vi "Configure Hardware r2.vi"(7 "DAQmx Cluster In":T1 {"ai DAQmx Cluster"."input terminal configuration" items=["Default"=-1, "RSE"=10083, "NRSE"=10078, "Differential"=10106, "Pseudodifferential"=12529]; "bc DAQmx Cluster"."Scaling Information"."electrical units" items=["Volts/Volt"=15896, "mVolts/Volt"=15897]; "bc DAQmx Cluster"."Scaling Information"."physical units" items=["Newtons"=15875, "Pounds"=15876, "kgf"=15877]; "bc DAQmx Cluster"."Bridge Information"."bridge configuration" items=["Full Bridge"=10182, "Half Bridge"=10187, "Quarter Bridge"=10270]; "bc DAQmx Cluster"."Bridge Information"."voltage excitation source" items=["Internal"=10200, "External"=10167]; "tc DAQmx Cluster"."Thermocouple Type" items=["J"=10072, "K"=10073, "N"=10077, "R"=10082, "S"=10085, "T"=10086, "B"=10047, "E"=10055]; "tc DAQmx Cluster"."Units" items=["Deg C"=10143, "Deg F"=10144, "Kelvins"=10325, "Deg R"=10145, "From Custom Scale"=10065]}, 8 "error in (no error)":errorcluster, 11 "DAQmx Container In":T2) -> (0 "error out":errorcluster, 3 "DAQmx Container Out":T2)   [LabVIEW 2024]
doc: "Configure the hardware."
uses:
  support/Control/DAQmx Container.ctl
  Configuration/DAQmx Configuration.ctl
  <vilib>/DAQmx/create/channels.llb/DAQmx Create Channel (DO-Digital Output).vi
  <vilib>/DAQmx/create/channels.llb/DAQmx Create Channel (AI-Force-Bridge-Two-Point-Linear).vi
  <vilib>/DAQmx/configure/timing.llb/DAQmx Timing (Sample Clock).vi
  <vilib>/DAQmx/create/channels.llb/DAQmx Create Channel (AI-Voltage-Basic).vi
  <vilib>/DAQmx/create/channels.llb/DAQmx Create Channel (AI-Temperature-Thermocouple).vi
  <vilib>/DAQmx/create/channels.llb/DAQmx Create Channel (DI-Digital Input).vi
  <resource>/objmgr/daqmx.rc
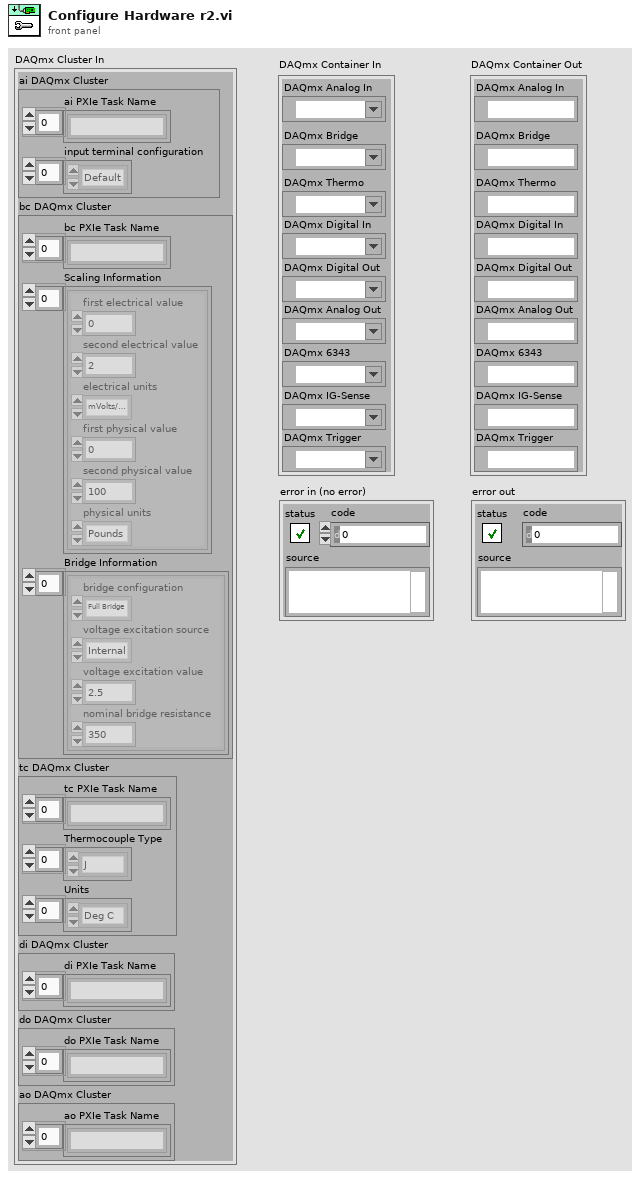
[diagram p1: front panel]
types:
  T1 = typedef "DAQmx Configuration.ctl" = cluster{"ai DAQmx Cluster":cluster{"ai PXIe Task Name":string[], "input terminal configuration":i32[]}, "bc DAQmx Cluster":cluster{"bc PXIe Task Name":string[], "Scaling Information":cluster{"first electrical value":dbl, "second electrical value":dbl, "electrical units":i32, "first physical value":dbl, "second physical value":dbl, "physical units":i32}[], "Bridge Information":cluster{"bridge configuration":i32, "voltage excitation source":i32, "voltage excitation value":dbl, "nominal bridge resistance":dbl}[]}, "tc DAQmx Cluster":cluster{"tc PXIe Task Name":string[], "Thermocouple Type":i32[], "Units":i32[]}, "di DAQmx Cluster":cluster{"di PXIe Task Name":string[]}, "do DAQmx Cluster":cluster{"do PXIe Task Name":string[]}, "ao DAQmx Cluster":cluster{"ao PXIe Task Name":string[]}}
  T2 = typedef "DAQmx Container.ctl" = cluster{"DAQmx Analog In":refnum<k21>, "DAQmx Digital In":refnum<k21>, "DAQmx Digital Out":refnum<k21>, "DAQmx Analog Out":refnum<k21>, "DAQmx 6343":refnum<k21>, "DAQmx IG-Sense":refnum<k21>, "DAQmx Thermo":refnum<k21>, "DAQmx Bridge":refnum<k21>, "DAQmx Trigger":refnum<k21>}
  T3 = cluster{"ai PXIe Task Name":string[], "input terminal configuration":i32[]}
  T4 = cluster{"bc PXIe Task Name":string[], "Scaling Information":cluster{"first electrical value":dbl, "second electrical value":dbl, "electrical units":i32, "first physical value":dbl, "second physical value":dbl, "physical units":i32}[], "Bridge Information":cluster{"bridge configuration":i32, "voltage excitation source":i32, "voltage excitation value":dbl, "nominal bridge resistance":dbl}[]}
  T5 = cluster{"tc PXIe Task Name":string[], "Thermocouple Type":i32[], "Units":i32[]}
  T6 = cluster{"bridge configuration":i32, "voltage excitation source":i32, "voltage excitation value":dbl, "nominal bridge resistance":dbl}[]
  T7 = cluster{"first electrical value":dbl, "second electrical value":dbl, "electrical units":i32, "first physical value":dbl, "second physical value":dbl, "physical units":i32}[]
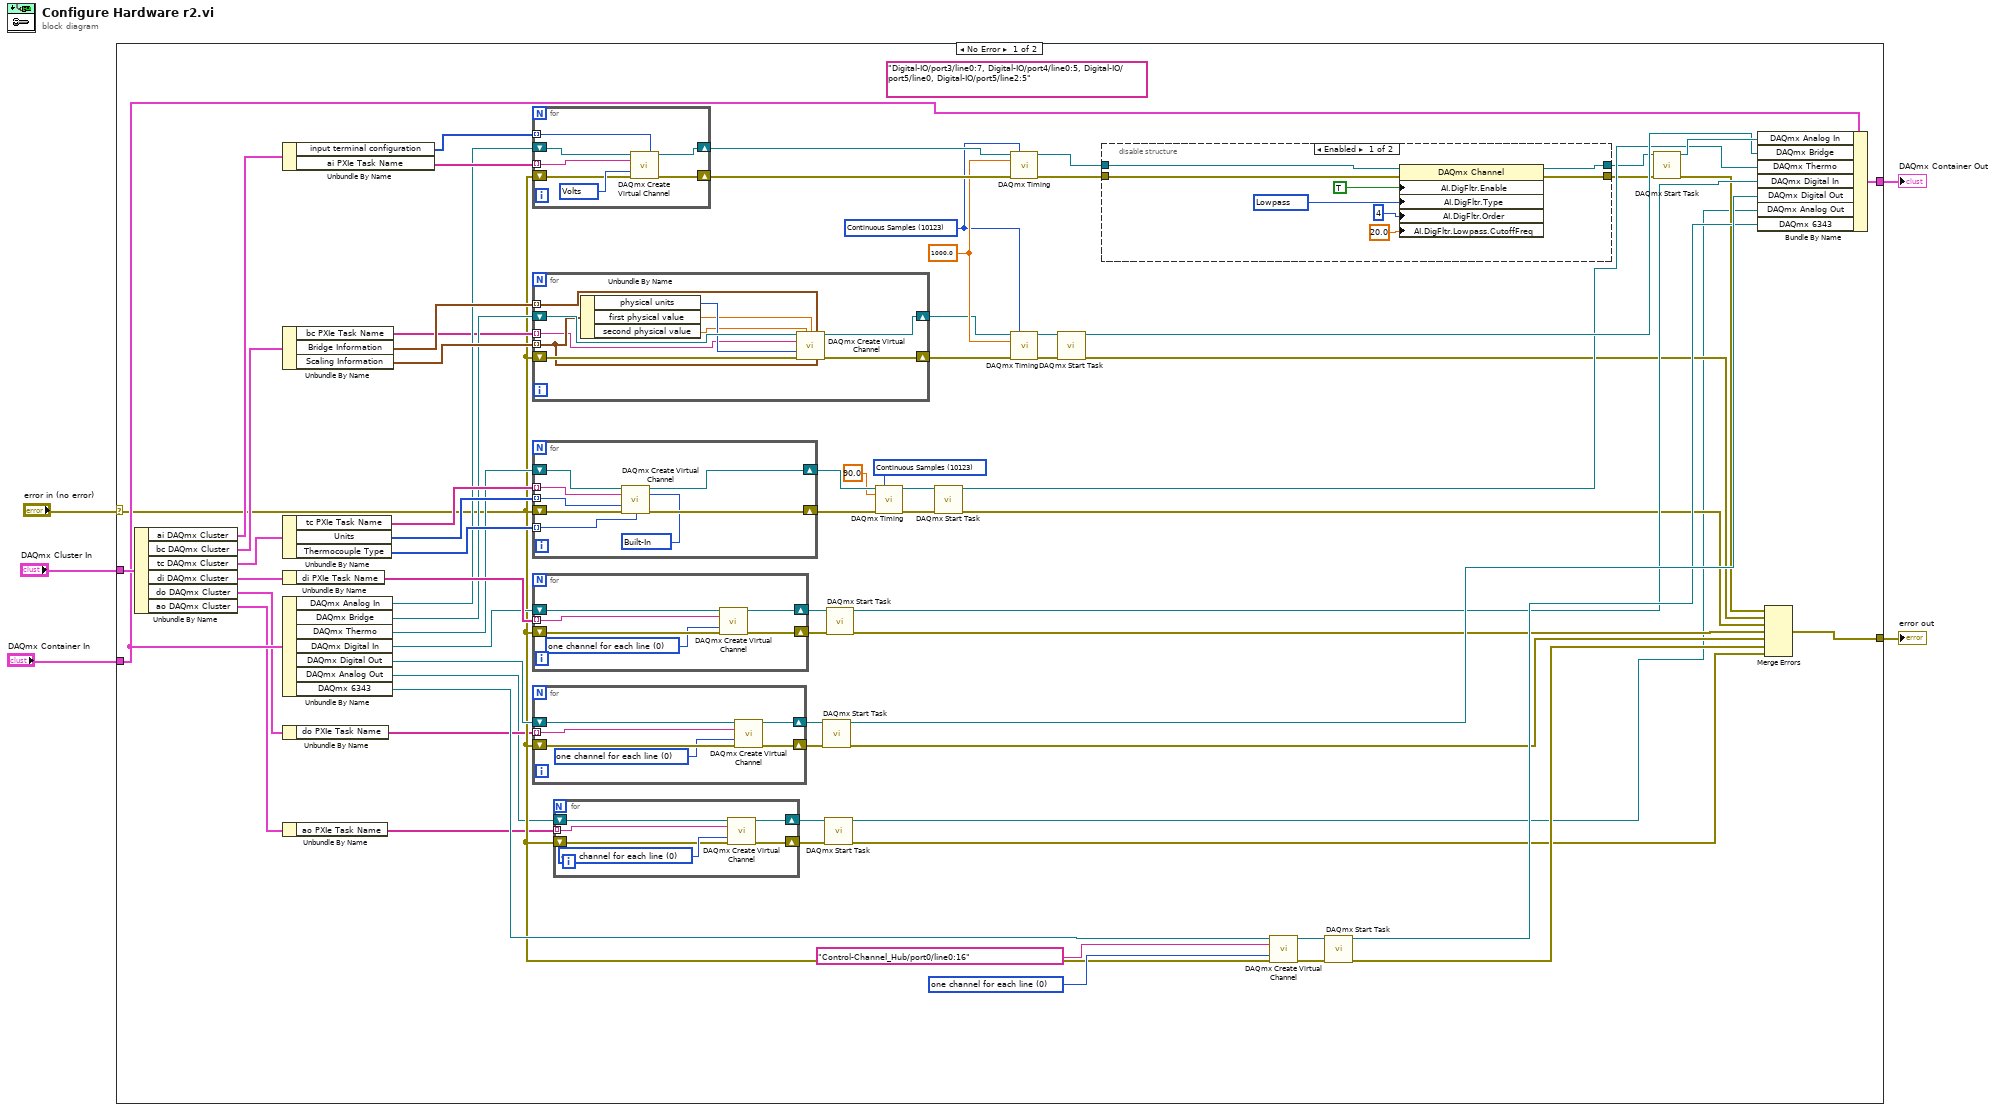
[diagram p0: block diagram]
diagram:
  n1 = case shown="No Error" "error in (no error)" {
    selector: "error in (no error)" -> [w10 w131]
    tunnel: [w30 w131] -> w4
    tunnel: [w29 w130] -> w3
    tunnel: "DAQmx Container In" -> [w55 w130]
    tunnel: "DAQmx Cluster In" -> [w76 _]
    frame No Error {
      (unwired) tag "Digital-IO/port3/line0:7, Digital-IO/port4/line0:5, Digital-IO/port5/line0, Digital-IO/port5/line2:5" ("lines")
      w42 = 10123 items=["Finite Samples"=10178, "Continuous Samples"=10123, "Hardware Timed Single Point"=12522] ("sample mode")
      w49 = 10123 items=["Finite Samples"=10178, "Continuous Samples"=10123, "Hardware Timed Single Point"=12522] ("sample mode")
      w50 = 1000.0 ("rate")
      w57 = 0 items=["one channel for each line", "one channel for all lines"] ("line grouping")
      n2 = Unbundle By Name(w76) -> ("ai DAQmx Cluster"=w75:T3, "bc DAQmx Cluster"=w72:T4, "tc DAQmx Cluster"=w69:T5, "di DAQmx Cluster"=w65:cluster{"di PXIe Task Name":string[]}, "do DAQmx Cluster"=w15:cluster{"do PXIe Task Name":string[]}, "ao DAQmx Cluster"=w14:cluster{"ao PXIe Task Name":string[]})
      n3 = Unbundle By Name(w75) -> ("input terminal configuration"=w73:i32[], "ai PXIe Task Name"=w74:string[])
      n4 = Unbundle By Name(w72) -> ("bc PXIe Task Name"=w20:string[], "Bridge Information"=w71:T6, "Scaling Information"=w70:T7)
      n5 = Unbundle By Name(w69) -> ("tc PXIe Task Name"=w66:string[], "Units"=w68:i32[], "Thermocouple Type"=w67:i32[])
      n6 = Unbundle By Name(w65) -> ("di PXIe Task Name"=w64:string[])
      n7 = Unbundle By Name(w55) -> ("DAQmx Analog In"=w63:refnum<k21>, "DAQmx Bridge"=w60:refnum<k21>, "DAQmx Thermo"=w62:refnum<k21>, "DAQmx Digital In"=w61:refnum<k21>, "DAQmx Digital Out"=w11:refnum<k21>, "DAQmx Analog Out"=w7:refnum<k21>, "DAQmx 6343"=w56:refnum<k21>)
      n8 = Unbundle By Name(w15) -> ("do PXIe Task Name"=w9:string[])
      n9 = Unbundle By Name(w14) -> ("ao PXIe Task Name"=w6:string[])
      n10 = for {
        tunnel: w74 -> [w129] mode=indexing
        tunnel: w73 -> [w128] mode=indexing
        shift-right: [w125] -> w52
        shift-left: w63 -> [w126]
        shift-right: [w124] -> w51
        shift-left: w10 -> [w123]
        w127 = 10348 items=["Volts"=10348, "From Custom Scale"=10065] ("units")
        n11 = call-poly <vilib>:"DAQmx Create Virtual Channel.vi"("task in"=w126, "input terminal configuration"=w128, "physical channels"=w129, "units"=w127, "error in"=w123) -> ("task out"=w125:refnum<k21>, "error out"=w124:errorcluster)  [unwired: 9 in]
      }
      n12 = for {
        shift-right: [w114] -> w19
        shift-left: w10 -> [w121]
        shift-right: [w115] -> w18
        shift-left: w60 -> [w122]
        tunnel: w20 -> [w113] mode=indexing
        tunnel: w71 -> [w120] mode=indexing
        tunnel: w70 -> [w119] mode=indexing
        n13 = Unbundle By Name(w119) -> ("physical units"=w118:i32, "first physical value"=w117:dbl, "second physical value"=w116:dbl)
        n14 = call-poly <vilib>:"DAQmx Create Virtual Channel.vi"("task in"=w122, "maximum value"=w116, "minimum value"=w117, "bridge information"=w120, "physical channels"=w113, "units"=w118, "error in"=w121, "scaling information"=w119) -> ("task out"=w115:refnum<k21>, "error out"=w114:errorcluster)  [unwired: 6 in]
      }
      n15 = for {
        shift-right: [w111] -> w44
        shift-left: w62 -> [w110]
        shift-right: [w112] -> w41
        shift-left: w10 -> [w107]
        tunnel: w68 -> [w105] mode=indexing
        tunnel: w67 -> [w106] mode=indexing
        tunnel: w66 -> [w108] mode=indexing
        w109 = 10200 items=["Built-In"=10200, "Constant Value"=10116, "Channel"=10113] ("cjc source")
        n16 = call-poly <vilib>:"DAQmx Create Virtual Channel.vi"("task in"=w110, "physical channels"=w108, "cjc source"=w109, "units"=w105, "error in"=w107, "thermocouple type"=w106) -> ("task out"=w111:refnum<k21>, "error out"=w112:errorcluster)  [unwired: 8 in]
      }
      n17 = for {
        shift-right: [w104] -> w46
        shift-left: w61 -> [w101]
        shift-right: [w103] -> w45
        shift-left: w10 -> [w102]
        tunnel: w64 -> [w100] mode=indexing
        w99 = 0 items=["one channel for each line", "one channel for all lines"] ("line grouping")
        n18 = call-poly <vilib>:"DAQmx Create Virtual Channel.vi"("task in"=w101, "lines"=w100, "line grouping"=w99, "error in"=w102) -> ("task out"=w104:refnum<k21>, "error out"=w103:errorcluster)  [unwired: 10 in]
      }
      n19 = for {
        shift-right: [w88] -> w13
        shift-left: w11 -> [w86]
        shift-right: [w87] -> w12
        shift-left: w10 -> [w85]
        tunnel: w9 -> [w83] mode=indexing
        w84 = 0 items=["one channel for each line", "one channel for all lines"] ("line grouping")
        n20 = call-poly <vilib>:"DAQmx Create Virtual Channel.vi"("task in"=w86, "lines"=w83, "line grouping"=w84, "error in"=w85) -> ("task out"=w88:refnum<k21>, "error out"=w87:errorcluster)  [unwired: 10 in]
      }
      n21 = for {
        shift-right: [w81] -> w23
        shift-left: w10 -> [w79]
        shift-right: [w80] -> w22
        shift-left: w7 -> [w78]
        tunnel: w6 -> [w77] mode=indexing
        w82 = 0 items=["one channel for each line", "one channel for all lines"] ("line grouping")
        n22 = call-poly <vilib>:"DAQmx Create Virtual Channel.vi"("task in"=w78, "lines"=w77, "line grouping"=w82, "error in"=w79) -> ("task out"=w80:refnum<k21>, "error out"=w81:errorcluster)  [unwired: 10 in]
      }
      n23 = call <vilib>:"DAQmx Start Task.vi"("task/channels in"=w13, "error in"=w12) -> ("task out"=w54:refnum<k21>, "error out"=w32:errorcluster)  [unwired: 12 in]
      n24 = call <vilib>:"DAQmx Start Task.vi"("task/channels in"=w22, "error in"=w23) -> ("task out"=w8:refnum<k21>, "error out"=w21:errorcluster)  [unwired: 12 in]
      n25 = call <vilib>:"DAQmx Start Task.vi"("task/channels in"=w46, "error in"=w45) -> ("task out"=w37:refnum<k21>, "error out"=w33:errorcluster)  [unwired: 12 in]
      n26 = call-poly <vilib>:"DAQmx Timing.vi"("task/channels in"=w44, "sample mode"=w42, "rate"=90.0, "error in"=w41) -> ("task out"=w40:refnum<k21>, "error out"=w39:errorcluster)  [unwired: 10 in]
      n27 = call <vilib>:"DAQmx Start Task.vi"("task/channels in"=w40, "error in"=w39) -> ("task out"=w38:refnum<k21>, "error out"=w34:errorcluster)  [unwired: 12 in]
      n28 = call-poly <vilib>:"DAQmx Timing.vi"("task/channels in"=w52, "sample mode"=w49, "rate"=w50, "error in"=w51) -> ("task out"=w27:refnum<k21>, "error out"=w25:errorcluster)  [unwired: 10 in]
      n29 = call-poly <vilib>:"DAQmx Timing.vi"("task/channels in"=w18, "sample mode"=w49, "rate"=w50, "error in"=w19) -> ("task out"=w17:refnum<k21>, "error out"=w16:errorcluster)  [unwired: 10 in]
      n30 = call <vilib>:"DAQmx Start Task.vi"("task/channels in"=w17, "error in"=w16) -> ("task out"=w47:refnum<k21>, "error out"=w35:errorcluster)  [unwired: 12 in]
      n31 = disable-structure shown="Enabled" {
        disable-tunnel: w27 -> [w96 w97]
        disable-tunnel: [w95 w97] -> w26
        disable-tunnel: w25 -> [w94 w98]
        disable-tunnel: [w93 w98] -> w24
        frame Enabled {
          w91 = 16071 items=["Lowpass"=16071, "Highpass"=16072, "Bandpass"=16073, "Notch"=16074, "Custom"=10137] ("AI.DigFltr.Type")
          n32 = property class="DAQmx Channel"(reference=w96, error in=w94, "AI.DigFltr.Enable"=TRUE, "AI.DigFltr.Type"=w91, "AI.DigFltr.Order"=u32 4, "AI.DigFltr.Lowpass.CutoffFreq"=20.0) -> (reference out=w95:refnum<k21>, error out=w93:errorcluster)
        }
        frame Disabled {
        }
      }
      n33 = call-poly <vilib>:"DAQmx Create Virtual Channel.vi"("task in"=w56, "lines"=tag "Control-Channel_Hub/port0/line0:16", "line grouping"=w57, "error in"=w10) -> ("task out"=w28:refnum<k21>, "error out"=w59:errorcluster)  [unwired: 10 in]
      n34 = call <vilib>:"DAQmx Start Task.vi"("task/channels in"=w28, "error in"=w59) -> ("task out"=w53:refnum<k21>, "error out"=w31:errorcluster)  [unwired: 12 in]
      n35 = call <vilib>:"DAQmx Start Task.vi"("task/channels in"=w26, "error in"=w24) -> ("task out"=w48:refnum<k21>, "error out"=w36:errorcluster)  [unwired: 12 in]
      n36 = Bundle By Name(cluster=w55, "DAQmx Analog In"=w48, "DAQmx Bridge"=w47, "DAQmx Thermo"=w38, "DAQmx Digital In"=w37, "DAQmx Digital Out"=w54, "DAQmx Analog Out"=w8, "DAQmx 6343"=w53) -> (w29:T2)
      n37 = Merge Errors(w36, w35, w34, w33, w32, w31, w21) -> (w30:errorcluster)
    }
    frame Error {
    }
  }
  "error out" <- w4
  "DAQmx Container Out" <- w3
